vi "加标回收调试界面.vi"() -> ()   [LabVIEW 2016, in "质控单元V4.lvlib"]
uses:
  <vilib>/Utility/miscctls.llb/LVPointTypeDef.ctl
panel:
  in  "关于":bool
  in  "关闭":bool
  in  "Tab Control 4":enum32{"参数"}(tab)
  out "剩余时间":string
  out "当前步骤":string
  out "当前流程":string
  out "告警状态":string
  out "液位状态":string
  out "运行状态":string
  in  "Tab Control 3":enum32{"单步调试", "流程控制"}(tab)
  in  "组合操作停止":bool
  in  "组合操作定量":bool
  in  "组合操作进空气":bool
  in  "组合操作排废液":bool
  in  "组合操作进水样":bool
  in  "蠕动泵2停止":bool
  in  "蠕动泵2正转":bool
  in  "蠕动泵2反转":bool
  in  "蠕动泵1停止":bool
  in  "蠕动泵1正转":bool
  in  "蠕动泵1反转":bool
  in  "三通阀2打开":bool
  in  "三通阀2关闭":bool
  in  "三通阀1打开":bool
  in  "三通阀1关闭":bool
  in  "注射泵复位":bool
  in  "注射泵暂停":bool
  in  "注射泵注入量":sgl
  in  "注射泵注出量":sgl
  in  "注射泵注出":bool
  in  "注射泵注入":bool
  in  "三通阀打开":bool
  in  "三通阀关闭":bool
  in  "清除告警":bool
  in  "停止所有流程":bool
  in  "启动排液流程":bool
  in  "启动加标流程":bool
  in  "启动进样流程":bool
  in  "启动润洗流程":bool
  in  "Tab Control 2":enum32{"参数"}(tab)
  in  "质控类型写入":bool
  in  "质控类型读取":bool
  in  "质控类型":u16(ring) items=["固定站", "一体站"]
  in  "注射泵系数写入":bool
  in  "注射泵系数读取":bool
  in  "加标体积(mL)":sgl
  in  "蠕动泵最大频率(Hz)":sgl
  in  "蠕动泵最小频率(Hz)":sgl
  in  "K":sgl
  in  "B":sgl
  in  "蠕动泵参数写入":bool
  in  "蠕动泵参数读取":bool
  in  "加标体积写入":bool
  in  "加标体积读取":bool
  in  "请选择模块":T1=enum."氨氮"
  # "仪器状态"
  # "柱塞泵"
  # "组合操作"
  # "三通阀"
  # "泵阀"
  # "三通阀1"
  # "三通阀2"
  # "蠕动泵1"
  # "蠕动泵2"
  # "参数设置"
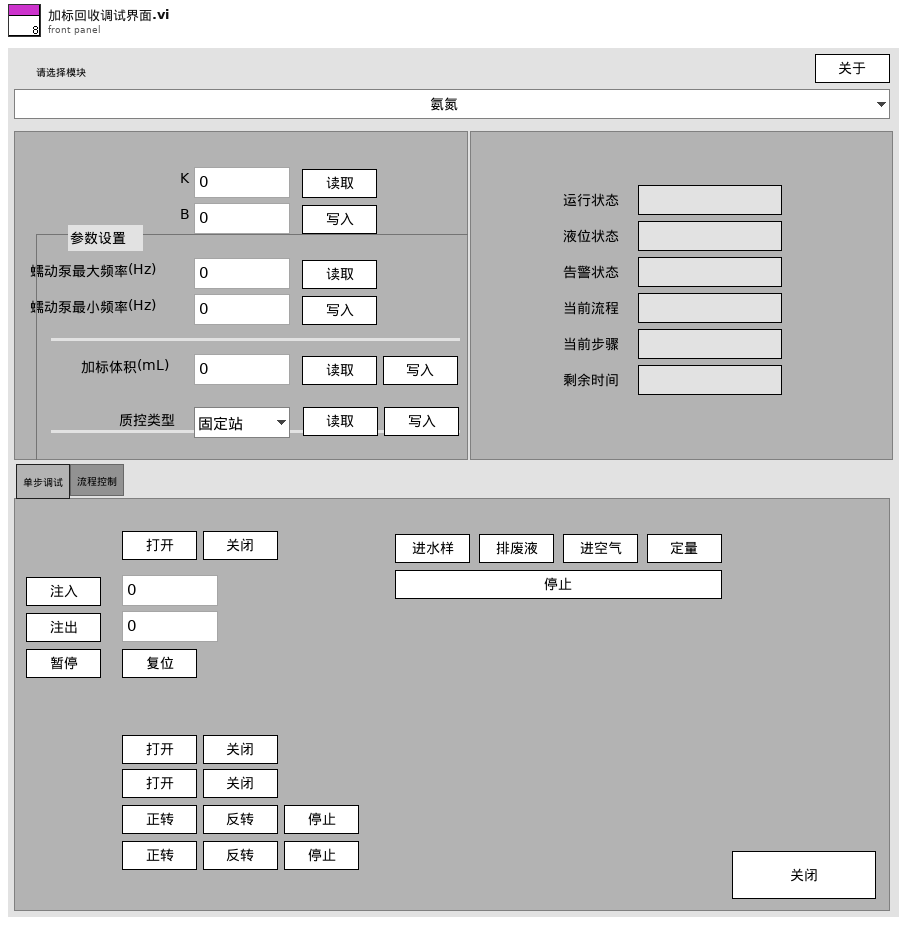
[diagram p1: front panel]
types:
  T1 = typedef "质控单元V4.lvlib/质控slave id.ctl" = enum16{"null", "氨氮", "总磷", "总氮", "CODMn", "CODCr", "氨氮总磷", "总磷总氮"}
  T2 = typedef "LVPointTypeDef.ctl" = cluster{"Horizontal":i16, "Vertical":i16}
  T3 = typedef "质控单元V4.lvlib/质控注射泵操作.ctl" = enum16{"打开三通阀", "关闭三通阀", "注射泵吸入", "注射泵排出", "注射泵暂停", "注射泵复位"}
  T4 = typedef "质控单元V4.lvlib/质控组合命令区.ctl" = enum16{"停止", "进水样", "排废液", "进空气（搅拌）", "定量（反转定量）"}
  T5 = typedef "质控单元V4.lvlib/质控流程控制.ctl" = enum16{"待机", "启动进样流程", "启动加标流程", "启动排液流程", "启动润洗流程", "停止流程"}
  T6 = typedef "质控单元V4.lvlib/质控仪器状态显示.ctl" = cluster{"运行状态":string, "液位状态":string, "告警状态":string, "当前流程":string, "当前步骤":string, "剩余时间":string}
  T7 = typedef "质控单元V4.lvlib/质控型号.ctl" = u16
  T8 = typedef "质控单元V4.lvlib/质控蠕动泵操作.ctl" = u16
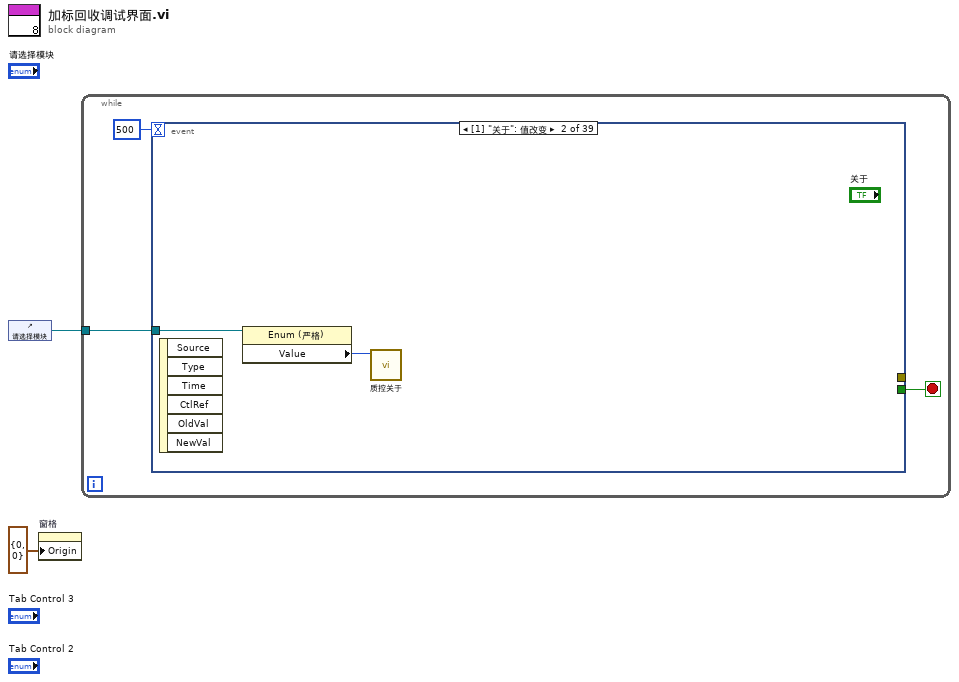
[diagram p0: block diagram]
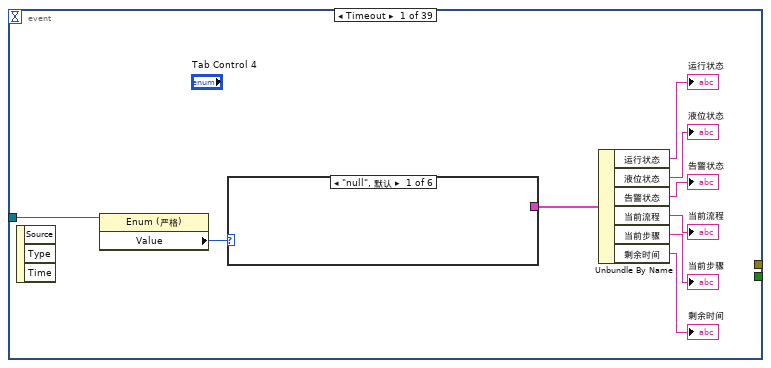
[diagram p2: hidden frame]
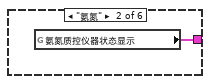
[diagram p3: hidden frame]
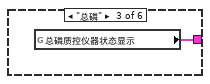
[diagram p4: hidden frame]
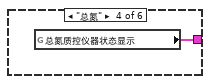
[diagram p5: hidden frame]
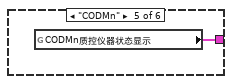
[diagram p6: hidden frame]
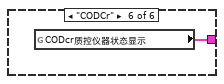
[diagram p7: hidden frame]
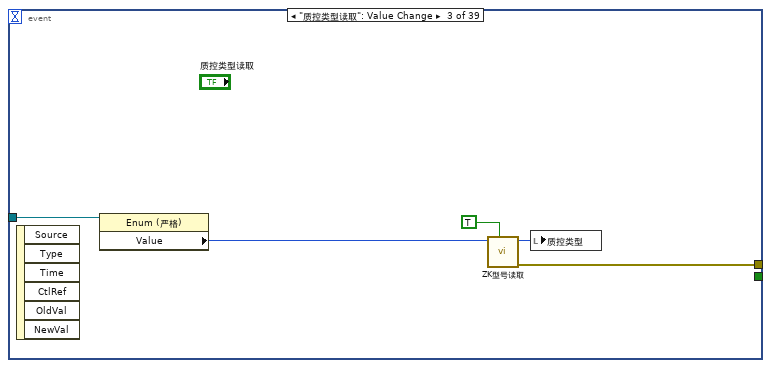
[diagram p8: hidden frame]
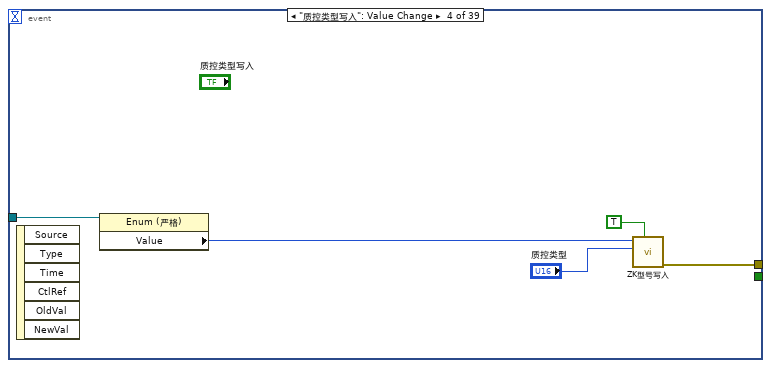
[diagram p9: hidden frame]
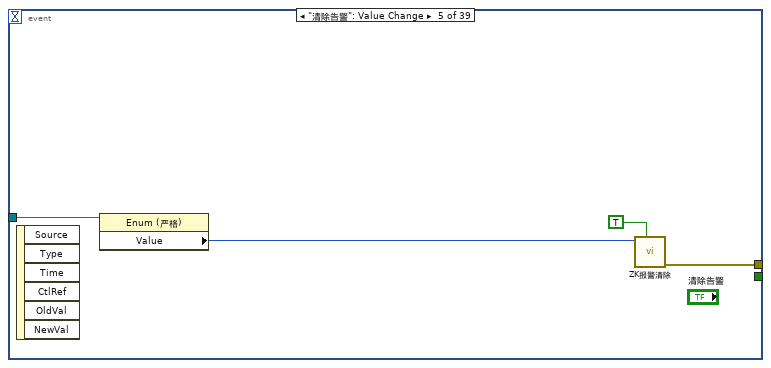
[diagram p10: hidden frame]
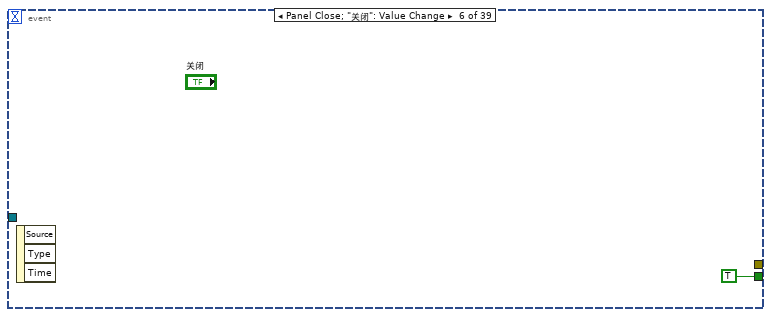
[diagram p11: hidden frame]
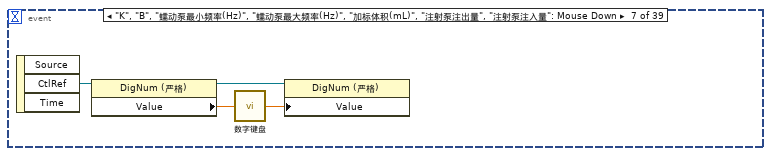
[diagram p12: hidden frame]
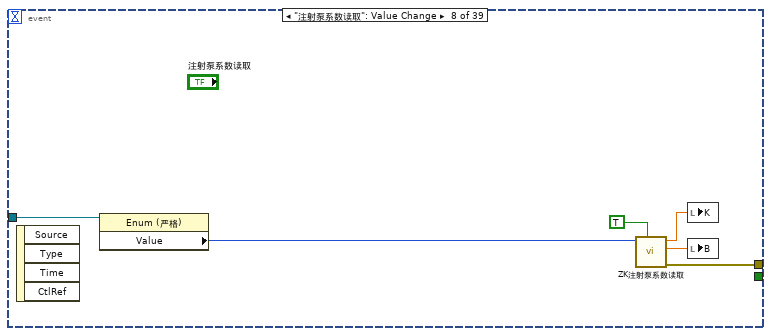
[diagram p13: hidden frame]
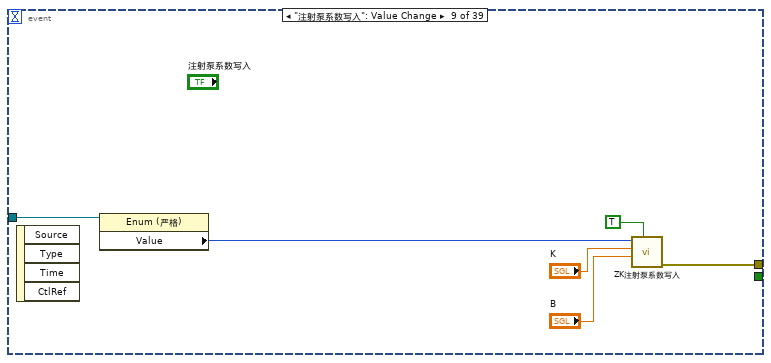
[diagram p14: hidden frame]
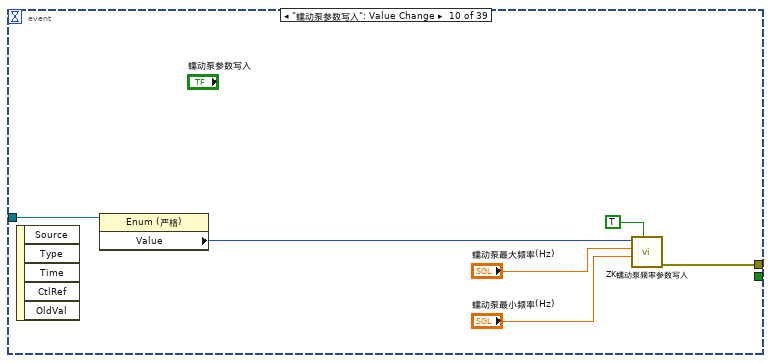
[diagram p15: hidden frame]
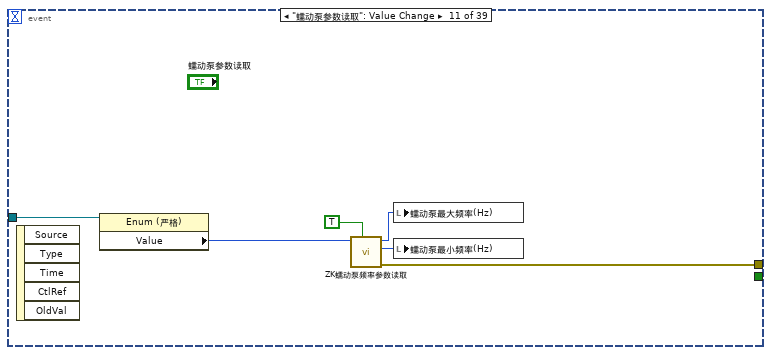
[diagram p16: hidden frame]
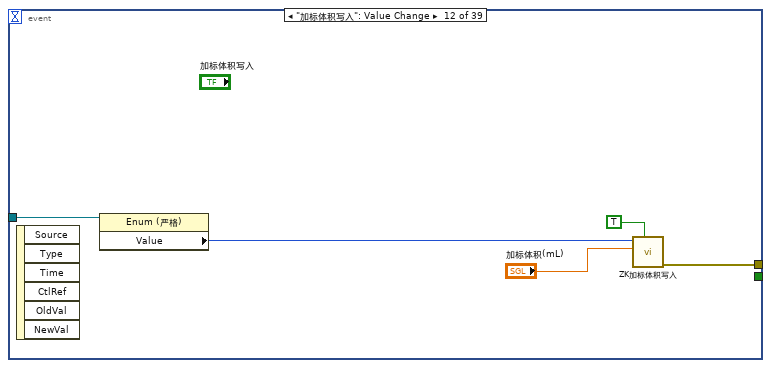
[diagram p17: hidden frame]
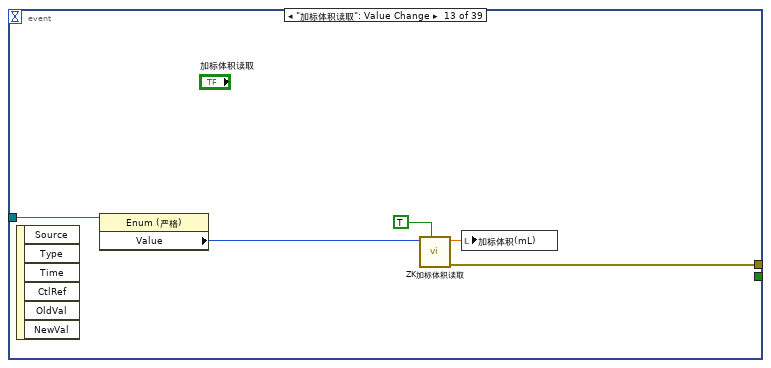
[diagram p18: hidden frame]
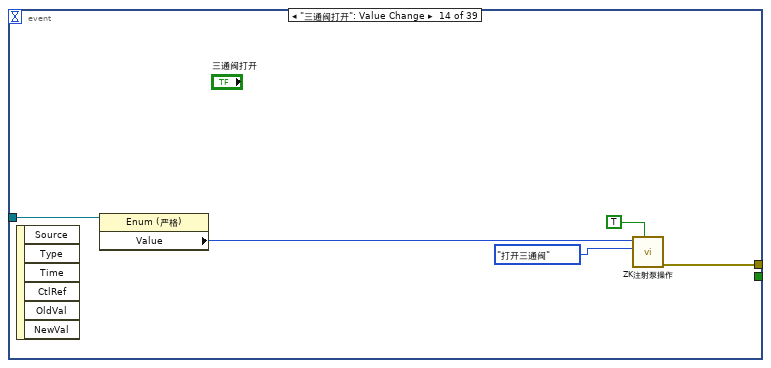
[diagram p19: hidden frame]
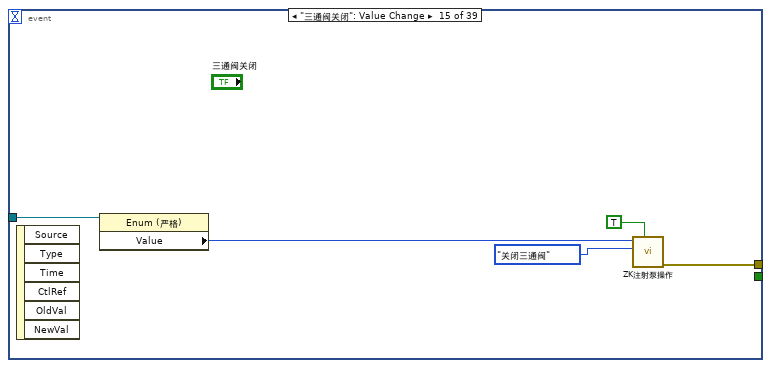
[diagram p20: hidden frame]
diagram:
  n1 = control-ref of="请选择模块"() -> (w1:refnum<vi>)
  n2 = property on="窗格" class="Pane"("Origin"=T2 {"Horizontal"=0, "Vertical"=0} ("原点")) -> ()  [unwired: 2 in, 2 out]
  n3 = while {
    tunnel: w1 -> [w4]
    stop <- w5 stop-if-true
    n4 = event shown="[1] \"关于\": 值改变" {
      selector: _ -> [_ _ _ _ _ _ _ _ _ _ _ _ _ _ _ _ _ _ _ _ _ _ _ _ _ _ _ _ _ _ _ _ _ _ _ _ _ _ _]
      dyn-events: _ -> [_ _ _ _ _ _ _ _ _ _ _ _ _ _ _ _ _ _ _ _ _ _ _ _ _ _ _ _ _ _ _ _ _ _ _ _ _ _ _]
      timeout: 500 -> [_ _ _ _ _ _ _ _ _ _ _ _ _ _ _ _ _ _ _ _ _ _ _ _ _ _ _ _ _ _ _ _ _ _ _ _ _ _ _]
      tunnel: [_ _ _ _ _ TRUE _ _ _ _ _ _ _ _ _ _ _ _ _ _ _ _ _ _ _ _ _ _ _ _ _ _ _ _ _ _ _ _ _] -> w5
      tunnel: w4 -> [w14 w21 w26 w31 w34 _ _ w46 w52 w58 w64 w67 w73 w78 w83 w90 w97 w102 w107 w111 w116 w123 w128 w131 w136 w141 w148 w153 w158 w162 w167 w172 w177 w182 w187 w192 w197 w202 w207]
      tunnel: [_ _ w22 w27 w35 _ _ w42 w48 w56 w60 w69 w74 w76 w84 w91 w98 w103 w108 w112 w117 w120 w125 w133 w138 w143 w146 w151 w156 w163 w168 w173 w178 w183 w188 w193 w198 w203 w208] -> _
      event Timeout {
        n5 = event-data() -> ()  [unwired: 1 in, 3 out]
        n6 = property class="Enum (严格)"(reference=w14) -> ("Value"=w13:T1)  [unwired: 1 in, 2 out]
        n7 = case shown="\"null\", 默认" w13 {
          tunnel: [_ w15 w16 w17 w18 w19] -> w12
          frame "null", Default {
          }
          frame "氨氮" {
            n8 = global read "ZK非断电保存全局变量.vi" "氨氮质控仪器状态显示"() -> (w15:T6)
          }
          frame "总磷" {
            n9 = global read "ZK非断电保存全局变量.vi" "总磷质控仪器状态显示"() -> (w16:T6)
          }
          frame "总氮" {
            n10 = global read "ZK非断电保存全局变量.vi" "总氮质控仪器状态显示"() -> (w17:T6)
          }
          frame "CODMn" {
            n11 = global read "ZK非断电保存全局变量.vi" "CODMn质控仪器状态显示"() -> (w18:T6)
          }
          frame "CODCr" {
            n12 = global read "ZK非断电保存全局变量.vi" "CODcr质控仪器状态显示"() -> (w19:T6)
          }
        }
        n13 = Unbundle By Name(w12) -> ("运行状态"=→"运行状态":string, "液位状态"=→"液位状态":string, "告警状态"=→"告警状态":string, "当前流程"=→"当前流程":string, "当前步骤"=→"当前步骤":string, "剩余时间"=→"剩余时间":string)
      }
      event "关于": Value Change {
        n14 = event-data() -> ()  [unwired: 1 in, 6 out]
        n15 = property class="Enum (严格)"(reference=w21) -> ("Value"=w20:T1)  [unwired: 1 in, 2 out]
        n16 = call "质控关于.vi"("Slave ID"=w20) -> ()  [unwired: 11 in]
      }
      event "质控类型读取": Value Change {
        n17 = event-data() -> ()  [unwired: 1 in, 6 out]
        n18 = property class="Enum (严格)"(reference=w26) -> ("Value"=w25:T1)  [unwired: 1 in, 2 out]
        n19 = call "ZK型号读取.vi"("是否启用通讯通知"=TRUE, "Slave ID"=w25) -> ("error out"=w22:errorcluster, "质控型号"=w23:T7)  [unwired: 8 in]
        n20 = local write "质控类型"(w23) -> ()
      }
      event "质控类型写入": Value Change {
        n21 = event-data() -> ()  [unwired: 1 in, 6 out]
        n22 = property class="Enum (严格)"(reference=w31) -> ("Value"=w30:T1)  [unwired: 1 in, 2 out]
        n23 = call "ZK型号写入.vi"("是否启用通讯通知"=TRUE, "质控型号"="质控类型", "Slave ID"=w30) -> ("error out"=w27:errorcluster)  [unwired: 8 in]
      }
      event "清除告警": Value Change {
        n24 = event-data() -> ()  [unwired: 1 in, 6 out]
        n25 = property class="Enum (严格)"(reference=w34) -> ("Value"=w33:T1)  [unwired: 1 in, 2 out]
        n26 = call "ZK报警清除.vi"("是否启用通讯通知"=TRUE, "Slave ID"=w33) -> ("error out"=w35:errorcluster)  [unwired: 9 in]
      }
      event Panel Close; "关闭": Value Change {
        n27 = event-data() -> ()  [unwired: 1 in, 3 out]
      }
      event "K", "B", "蠕动泵最小频率(Hz)", "蠕动泵最大频率(Hz)", "加标体积(mL)", "注射泵注出量", "注射泵注入量": Mouse Down {
        n28 = event-data() -> ("CtlRef"=w40:refnum<vi>)  [unwired: 1 in, 2 out]
        n29 = property class="DigNum (严格)"(reference=w40) -> (reference out=w38:refnum<vi>, "Value"=w39:sgl)  [unwired: 1 in, 1 out]
        n30 = call "数字键盘.vi"("OldNumber"=w39) -> ("NewNumber"=w37:sgl)
        n31 = property class="DigNum (严格)"(reference=w38, "Value"=w37) -> ()  [unwired: 1 in, 2 out]
      }
      event "注射泵系数读取": Value Change {
        n32 = event-data() -> ()  [unwired: 1 in, 4 out]
        n33 = property class="Enum (严格)"(reference=w46) -> ("Value"=w45:T1)  [unwired: 1 in, 2 out]
        n34 = call "ZK注射泵系数读取.vi"("是否启用通讯通知"=TRUE, "Slave ID"=w45) -> ("error out"=w42:errorcluster, "B"=w43:sgl, "K"=w44:sgl)  [unwired: 7 in]
        n35 = local write "K"(w44) -> ()
        n36 = local write "B"(w43) -> ()
      }
      event "注射泵系数写入": Value Change {
        n37 = event-data() -> ()  [unwired: 1 in, 4 out]
        n38 = property class="Enum (严格)"(reference=w52) -> ("Value"=w51:T1)  [unwired: 1 in, 2 out]
        n39 = call "ZK注射泵系数写入.vi"("是否启用通讯通知"=TRUE, "B"="B", "K"="K", "Slave ID"=w51) -> ("error out"=w48:errorcluster)  [unwired: 7 in]
      }
      event "蠕动泵参数写入": Value Change {
        n40 = event-data() -> ()  [unwired: 1 in, 5 out]
        n41 = property class="Enum (严格)"(reference=w58) -> ("Value"=w57:T1)  [unwired: 1 in, 2 out]
        n42 = call "ZK蠕动泵频率参数写入.vi"("是否启用通讯通知"=TRUE, "蠕动泵最小频率"="蠕动泵最小频率(Hz)", "蠕动泵最大频率"="蠕动泵最大频率(Hz)", "Slave ID"=w57) -> ("error out"=w56:errorcluster)  [unwired: 7 in]
      }
      event "蠕动泵参数读取": Value Change {
        n43 = event-data() -> ()  [unwired: 1 in, 5 out]
        n44 = property class="Enum (严格)"(reference=w64) -> ("Value"=w63:T1)  [unwired: 1 in, 2 out]
        n45 = call "ZK蠕动泵频率参数读取.vi"("是否启用通讯通知"=TRUE, "Slave ID"=w63) -> ("error out"=w60:errorcluster, "蠕动泵最小频率"=w61:i32, "蠕动泵最大频率"=w62:i32)  [unwired: 7 in]
        n46 = local write "蠕动泵最大频率(Hz)"(w62) -> ()
        n47 = local write "蠕动泵最小频率(Hz)"(w61) -> ()
      }
      event "加标体积写入": Value Change {
        n48 = event-data() -> ()  [unwired: 1 in, 6 out]
        n49 = property class="Enum (严格)"(reference=w67) -> ("Value"=w66:T1)  [unwired: 1 in, 2 out]
        n50 = call "ZK加标体积写入.vi"("是否启用通讯通知"=TRUE, "加标体积"="加标体积(mL)", "Slave ID"=w66) -> ("error out"=w69:errorcluster)  [unwired: 8 in]
      }
      event "加标体积读取": Value Change {
        n51 = event-data() -> ()  [unwired: 1 in, 6 out]
        n52 = property class="Enum (严格)"(reference=w73) -> ("Value"=w72:T1)  [unwired: 1 in, 2 out]
        n53 = call "ZK加标体积读取.vi"("是否启用通讯通知"=TRUE, "Slave ID"=w72) -> ("error out"=w74:errorcluster, "加标体积"=w71:sgl)  [unwired: 8 in]
        n54 = local write "加标体积(mL)"(w71) -> ()
      }
      event "三通阀打开": Value Change {
        n55 = event-data() -> ()  [unwired: 1 in, 6 out]
        n56 = property class="Enum (严格)"(reference=w78) -> ("Value"=w77:T1)  [unwired: 1 in, 2 out]
        n57 = call "ZK注射泵操作.vi"("是否启用通讯通知"=TRUE, "注射泵操作"=质控注射泵操作."打开三通阀", "Slave ID"=w77) -> ("error out"=w76:errorcluster)  [unwired: 8 in]
      }
      event "三通阀关闭": Value Change {
        n58 = event-data() -> ()  [unwired: 1 in, 6 out]
        n59 = property class="Enum (严格)"(reference=w83) -> ("Value"=w82:T1)  [unwired: 1 in, 2 out]
        n60 = call "ZK注射泵操作.vi"("是否启用通讯通知"=TRUE, "注射泵操作"=质控注射泵操作."关闭三通阀", "Slave ID"=w82) -> ("error out"=w84:errorcluster)  [unwired: 8 in]
      }
      event "注射泵注入": Value Change {
        n61 = event-data() -> ()  [unwired: 1 in, 6 out]
        n62 = property class="Enum (严格)"(reference=w90) -> ("Value"=w87:T1)  [unwired: 1 in, 2 out]
        n63 = call "ZK注射泵操作步.vi"("注射泵操作步"="注射泵注入量", "Slave ID"=w87) -> ("error out"=w88:errorcluster)  [unwired: 9 in]
        n64 = call "ZK注射泵操作.vi"("是否启用通讯通知"=TRUE, "error in (no error)"=w88, "注射泵操作"=质控注射泵操作."注射泵吸入", "Slave ID"=w87) -> ("error out"=w91:errorcluster)  [unwired: 7 in]
      }
      event "注射泵注出": Value Change {
        n65 = event-data() -> ()  [unwired: 1 in, 6 out]
        n66 = property class="Enum (严格)"(reference=w97) -> ("Value"=w94:T1)  [unwired: 1 in, 2 out]
        n67 = call "ZK注射泵操作步.vi"("注射泵操作步"="注射泵注出量", "Slave ID"=w94) -> ("error out"=w95:errorcluster)  [unwired: 9 in]
        n68 = call "ZK注射泵操作.vi"("是否启用通讯通知"=TRUE, "error in (no error)"=w95, "注射泵操作"=质控注射泵操作."注射泵排出", "Slave ID"=w94) -> ("error out"=w98:errorcluster)  [unwired: 7 in]
      }
      event "注射泵暂停": Value Change {
        n69 = event-data() -> ()  [unwired: 1 in, 6 out]
        n70 = property class="Enum (严格)"(reference=w102) -> ("Value"=w100:T1)  [unwired: 1 in, 2 out]
        n71 = call "ZK注射泵操作.vi"("是否启用通讯通知"=TRUE, "注射泵操作"=质控注射泵操作."注射泵暂停", "Slave ID"=w100) -> ("error out"=w103:errorcluster)  [unwired: 8 in]
      }
      event "注射泵复位": Value Change {
        n72 = event-data() -> ()  [unwired: 1 in, 6 out]
        n73 = property class="Enum (严格)"(reference=w107) -> ("Value"=w105:T1)  [unwired: 1 in, 2 out]
        n74 = call "ZK注射泵操作.vi"("是否启用通讯通知"=TRUE, "注射泵操作"=质控注射泵操作."注射泵复位", "Slave ID"=w105) -> ("error out"=w108:errorcluster)  [unwired: 8 in]
      }
      event "三通阀1关闭": Value Change {
        w113 = u16 1 items=["打开三通阀", "关闭三通阀"] ("三通阀1操作")
        n75 = event-data() -> ()  [unwired: 1 in, 6 out]
        n76 = property class="Enum (严格)"(reference=w111) -> ("Value"=w110:T1)  [unwired: 1 in, 2 out]
        n77 = call "ZK三通阀1操作.vi"("是否启用通讯通知"=TRUE, "三通阀1操作"=w113, "Slave ID"=w110) -> ("error out"=w112:errorcluster)  [unwired: 8 in]
      }
      event "三通阀1打开": Value Change {
        w118 = u16 0 items=["打开三通阀", "关闭三通阀"] ("三通阀1操作")
        n78 = event-data() -> ()  [unwired: 1 in, 6 out]
        n79 = property class="Enum (严格)"(reference=w116) -> ("Value"=w115:T1)  [unwired: 1 in, 2 out]
        n80 = call "ZK三通阀1操作.vi"("是否启用通讯通知"=TRUE, "三通阀1操作"=w118, "Slave ID"=w115) -> ("error out"=w117:errorcluster)  [unwired: 8 in]
      }
      event "三通阀2打开": Value Change {
        w121 = u16 0 items=["打开三通阀", "关闭三通阀"] ("三通阀2操作")
        n81 = event-data() -> ()  [unwired: 1 in, 6 out]
        n82 = property class="Enum (严格)"(reference=w123) -> ("Value"=w122:T1)  [unwired: 1 in, 2 out]
        n83 = call "ZK三通阀2操作.vi"("是否启用通讯通知"=TRUE, "三通阀2操作"=w121, "Slave ID"=w122) -> ("error out"=w120:errorcluster)  [unwired: 8 in]
      }
      event "三通阀2关闭": Value Change {
        w126 = u16 1 items=["打开三通阀", "关闭三通阀"] ("三通阀2操作")
        n84 = event-data() -> ()  [unwired: 1 in, 6 out]
        n85 = property class="Enum (严格)"(reference=w128) -> ("Value"=w127:T1)  [unwired: 1 in, 2 out]
        n86 = call "ZK三通阀2操作.vi"("是否启用通讯通知"=TRUE, "三通阀2操作"=w126, "Slave ID"=w127) -> ("error out"=w125:errorcluster)  [unwired: 8 in]
      }
      event "蠕动泵1反转": Value Change {
        w132 = T8 3 items=["蠕动泵正转"=2, "蠕动泵反转"=3, "蠕动泵停止"=4] ("蠕动泵1操作")
        n87 = event-data() -> ()  [unwired: 1 in, 6 out]
        n88 = property class="Enum (严格)"(reference=w131) -> ("Value"=w130:T1)  [unwired: 1 in, 2 out]
        n89 = call "ZK蠕动泵1操作.vi"("是否启用通讯通知"=TRUE, "蠕动泵1操作"=w132, "Slave ID"=w130) -> ("error out"=w133:errorcluster)  [unwired: 8 in]
      }
      event "蠕动泵1正转": Value Change {
        w137 = T8 2 items=["蠕动泵正转"=2, "蠕动泵反转"=3, "蠕动泵停止"=4] ("蠕动泵1操作")
        n90 = event-data() -> ()  [unwired: 1 in, 6 out]
        n91 = property class="Enum (严格)"(reference=w136) -> ("Value"=w135:T1)  [unwired: 1 in, 2 out]
        n92 = call "ZK蠕动泵1操作.vi"("是否启用通讯通知"=TRUE, "蠕动泵1操作"=w137, "Slave ID"=w135) -> ("error out"=w138:errorcluster)  [unwired: 8 in]
      }
      event "蠕动泵1停止": Value Change {
        w142 = T8 4 items=["蠕动泵正转"=2, "蠕动泵反转"=3, "蠕动泵停止"=4] ("蠕动泵1操作")
        n93 = event-data() -> ()  [unwired: 1 in, 6 out]
        n94 = property class="Enum (严格)"(reference=w141) -> ("Value"=w140:T1)  [unwired: 1 in, 2 out]
        n95 = call "ZK蠕动泵1操作.vi"("是否启用通讯通知"=TRUE, "蠕动泵1操作"=w142, "Slave ID"=w140) -> ("error out"=w143:errorcluster)  [unwired: 8 in]
      }
      event "蠕动泵2反转": Value Change {
        w145 = T8 3 items=["蠕动泵正转"=2, "蠕动泵反转"=3, "蠕动泵停止"=4] ("蠕动泵2操作")
        n96 = event-data() -> ()  [unwired: 1 in, 6 out]
        n97 = property class="Enum (严格)"(reference=w148) -> ("Value"=w147:T1)  [unwired: 1 in, 2 out]
        n98 = call "ZK蠕动泵2操作.vi"("是否启用通讯通知"=TRUE, "蠕动泵2操作"=w145, "Slave ID"=w147) -> ("error out"=w146:errorcluster)  [unwired: 8 in]
      }
      event "蠕动泵2正转": Value Change {
        w150 = T8 2 items=["蠕动泵正转"=2, "蠕动泵反转"=3, "蠕动泵停止"=4] ("蠕动泵2操作")
        n99 = event-data() -> ()  [unwired: 1 in, 6 out]
        n100 = property class="Enum (严格)"(reference=w153) -> ("Value"=w152:T1)  [unwired: 1 in, 2 out]
        n101 = call "ZK蠕动泵2操作.vi"("是否启用通讯通知"=TRUE, "蠕动泵2操作"=w150, "Slave ID"=w152) -> ("error out"=w151:errorcluster)  [unwired: 8 in]
      }
      event "蠕动泵2停止": Value Change {
        w155 = T8 4 items=["蠕动泵正转"=2, "蠕动泵反转"=3, "蠕动泵停止"=4] ("蠕动泵2操作")
        n102 = event-data() -> ()  [unwired: 1 in, 6 out]
        n103 = property class="Enum (严格)"(reference=w158) -> ("Value"=w157:T1)  [unwired: 1 in, 2 out]
        n104 = call "ZK蠕动泵2操作.vi"("是否启用通讯通知"=TRUE, "蠕动泵2操作"=w155, "Slave ID"=w157) -> ("error out"=w156:errorcluster)  [unwired: 8 in]
      }
      event "组合操作进水样": Value Change {
        n105 = event-data() -> ()  [unwired: 1 in, 6 out]
        n106 = property class="Enum (严格)"(reference=w162) -> ("Value"=w161:T1)  [unwired: 1 in, 2 out]
        n107 = call "ZK组合命令区.vi"("是否启用通讯通知"=TRUE, "组合命令区"=质控组合命令区."进水样", "Slave ID"=w161) -> ("error out"=w163:errorcluster)  [unwired: 8 in]
      }
      event "组合操作排废液": Value Change {
        n108 = event-data() -> ()  [unwired: 1 in, 6 out]
        n109 = property class="Enum (严格)"(reference=w167) -> ("Value"=w166:T1)  [unwired: 1 in, 2 out]
        n110 = call "ZK组合命令区.vi"("是否启用通讯通知"=TRUE, "组合命令区"=质控组合命令区."排废液", "Slave ID"=w166) -> ("error out"=w168:errorcluster)  [unwired: 8 in]
      }
      event "组合操作进空气": Value Change {
        n111 = event-data() -> ()  [unwired: 1 in, 6 out]
        n112 = property class="Enum (严格)"(reference=w172) -> ("Value"=w171:T1)  [unwired: 1 in, 2 out]
        n113 = call "ZK组合命令区.vi"("是否启用通讯通知"=TRUE, "组合命令区"=质控组合命令区."进空气（搅拌）", "Slave ID"=w171) -> ("error out"=w173:errorcluster)  [unwired: 8 in]
      }
      event "组合操作定量": Value Change {
        n114 = event-data() -> ()  [unwired: 1 in, 6 out]
        n115 = property class="Enum (严格)"(reference=w177) -> ("Value"=w176:T1)  [unwired: 1 in, 2 out]
        n116 = call "ZK组合命令区.vi"("是否启用通讯通知"=TRUE, "组合命令区"=质控组合命令区."定量（反转定量）", "Slave ID"=w176) -> ("error out"=w178:errorcluster)  [unwired: 8 in]
      }
      event "组合操作停止": Value Change {
        n117 = event-data() -> ()  [unwired: 1 in, 6 out]
        n118 = property class="Enum (严格)"(reference=w182) -> ("Value"=w181:T1)  [unwired: 1 in, 2 out]
        n119 = call "ZK组合命令区.vi"("是否启用通讯通知"=TRUE, "组合命令区"=质控组合命令区."停止", "Slave ID"=w181) -> ("error out"=w183:errorcluster)  [unwired: 8 in]
      }
      event "启动进样流程": Value Change {
        n120 = event-data() -> ()  [unwired: 1 in, 6 out]
        n121 = property class="Enum (严格)"(reference=w187) -> ("Value"=w186:T1)  [unwired: 1 in, 2 out]
        n122 = call "ZK流程控制.vi"("是否启用通讯通知"=TRUE, "流程控制"=质控流程控制."启动进样流程", "Slave ID"=w186) -> ("error out"=w188:errorcluster)  [unwired: 8 in]
      }
      event "启动加标流程": Value Change {
        n123 = event-data() -> ()  [unwired: 1 in, 6 out]
        n124 = property class="Enum (严格)"(reference=w192) -> ("Value"=w191:T1)  [unwired: 1 in, 2 out]
        n125 = call "ZK流程控制.vi"("是否启用通讯通知"=TRUE, "流程控制"=质控流程控制."启动加标流程", "Slave ID"=w191) -> ("error out"=w193:errorcluster)  [unwired: 8 in]
      }
      event "启动排液流程": Value Change {
        n126 = event-data() -> ()  [unwired: 1 in, 6 out]
        n127 = property class="Enum (严格)"(reference=w197) -> ("Value"=w196:T1)  [unwired: 1 in, 2 out]
        n128 = call "ZK流程控制.vi"("是否启用通讯通知"=TRUE, "流程控制"=质控流程控制."启动排液流程", "Slave ID"=w196) -> ("error out"=w198:errorcluster)  [unwired: 8 in]
      }
      event "停止所有流程": Value Change {
        n129 = event-data() -> ()  [unwired: 1 in, 6 out]
        n130 = property class="Enum (严格)"(reference=w202) -> ("Value"=w201:T1)  [unwired: 1 in, 2 out]
        n131 = call "ZK流程控制.vi"("是否启用通讯通知"=TRUE, "流程控制"=质控流程控制."停止流程", "Slave ID"=w201) -> ("error out"=w203:errorcluster)  [unwired: 8 in]
      }
      event "启动润洗流程": Value Change {
        n132 = event-data() -> ()  [unwired: 1 in, 6 out]
        n133 = property class="Enum (严格)"(reference=w207) -> ("Value"=w206:T1)  [unwired: 1 in, 2 out]
        n134 = call "ZK流程控制.vi"("是否启用通讯通知"=TRUE, "流程控制"=质控流程控制."启动润洗流程", "Slave ID"=w206) -> ("error out"=w208:errorcluster)  [unwired: 8 in]
      }
    }
  }
